vi "Test Name of Test Case in Result when Creating Suite from Test Case.vi"(8 "error in (no error)":errorcluster, 11 "Test Case In":refnum<class "LUnit Test Suite Tests.lvclass">) -> (0 "error out":errorcluster, 3 "Test Case Out":refnum<class "LUnit Test Suite Tests.lvclass">)   [LabVIEW 2020, in "LUnit Test Suite Tests.lvclass"]
uses:
  LUnit Test Suite Tests.lvclass
  LUnit Test Suite Tests.lvclass/LUnit Test Suite Tests.ctl
  b74e4934-f044-4222-b3dd-fc90e6c1bd4f.vi
  Test Doubles/Test Case Test Double/Test Case Test Double.lvclass
  source/LUnit Test Suite.lvclass
  C:/git/astemes-lunit/source/Core/Runnable/Runnable.lvclass
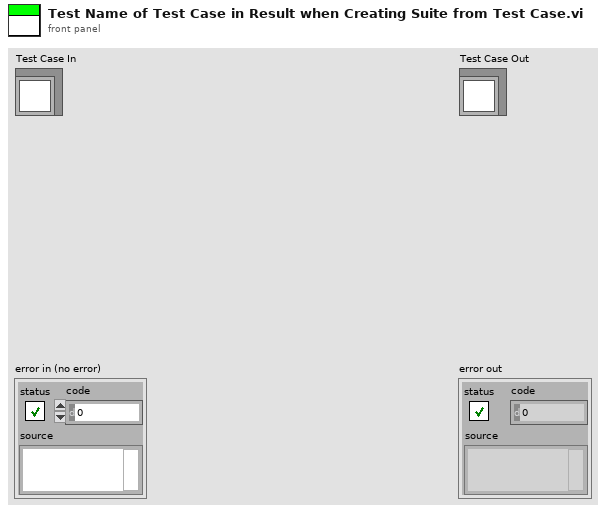
[diagram p1: front panel]
types:
  T1 = typedef "Result.lvlib/Result.ctl" = cluster{"Name":string, "Description":string, "Status":T2, "Result Type":T3, "Execution Time":dbl, "Data":cluster{"Expected":variant, "Actual":variant, "Delta":variant}}
  T2 = typedef "Result.lvlib/Status.ctl" = enum16{"", "Passed", "Failed", "Error", "Skipped", "Setup Error", "Broken", "Teardown Error"}
  T3 = typedef "Result.lvlib/Type.ctl" = enum16{"Test Case", "Test Suite", "Test Run", "Pass", "Fail", "Skip", "Pass if", "Fail if", "Pass if Error", "Fail if Error", "Pass if Equal", "Fail if Equal"}
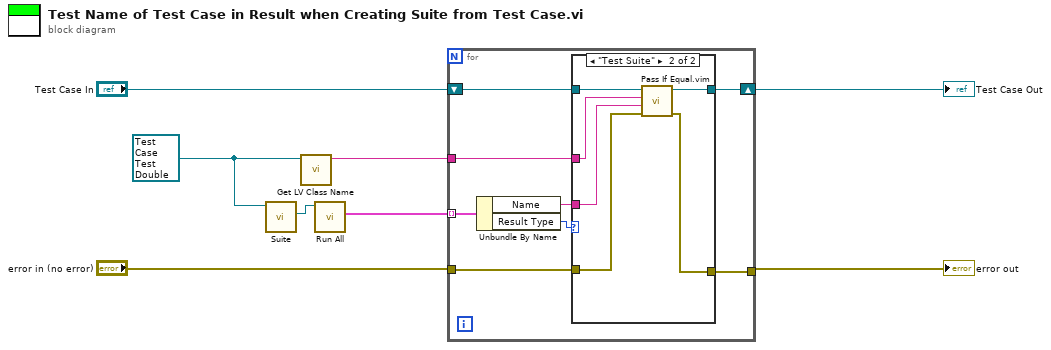
[diagram p0: block diagram]
diagram:
  w7 = refnum<class "Test Case Test Double.lvclass"> refnum ("LUnit Test Case V2 Test Double.lvclass")
  n1 = call-dynamic "Suite.vi"("LUnit Test Case In"=w7) -> ("LUnit Test Suite Out"=w8:refnum<class "LUnit Test Suite.lvclass">)  [unwired: 8 in, 2 out]
  n2 = call <vilib>:"Get LV Class Name.vi"("object"=w7) -> ("class name"=w1:string)  [unwired: 9 in, 1 out]
  n3 = call "Run All.vi"("Runnable In"=w8) -> ("Results"=w6:T1[])  [unwired: 9 in, 1 out]
  n4 = for {
    tunnel: w6 -> [w16] mode=indexing
    tunnel: "error in (no error)" -> [w15]
    tunnel: [w13] -> w3
    shift-right: [w12] -> w2
    shift-left: "Test Case In" -> [w14]
    tunnel: w1 -> [w11]
    n5 = Unbundle By Name(w16) -> ("Name"=w10:string, "Result Type"=w9:T3)
    n6 = case shown="\"Test Suite\"" w9 {
      tunnel: w15 -> [w17 w24]
      tunnel: w14 -> [w18 w23]
      tunnel: [w17 w22] -> w13
      tunnel: [w18 w21] -> w12
      tunnel: w11 -> [_ w20]
      tunnel: w10 -> [_ w19]
      frame Default {
      }
      frame "Test Suite" {
        n7 = call "Pass If Equal.vim"("error in (no error)"=w24, "Actual"=w19, "Expected"=w20, "LUnit Test Case In"=w23) -> ("error out"=w22:errorcluster, "LUnit Test Case Out"=w21:refnum<class "LUnit Test Suite Tests.lvclass">)  [unwired: 6 in]
      }
    }
  }
  "error out" <- w3
  "Test Case Out" <- w2
